vi "Read-Only Globals.vi"() -> (2 "Round":i32, 3 "Board Size":i32)   [LabVIEW 2020, in "SB SubVIs.lvlib"]
uses:
  SB SubVIs.lvlib
  Globals (private).vi
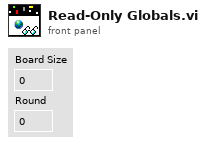
[diagram p1: front panel]
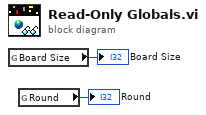
[diagram p0: block diagram]
diagram:
  n1 = global read "Globals (private).vi" "Board Size"() -> (→"Board Size":i32)
  n2 = global read "Globals (private).vi" "Round"() -> (→"Round":i32)
